vi "LCd.vi"() -> ()   [LabVIEW 2017]
panel:
  in  "String":string
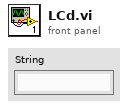
[diagram p1: front panel]
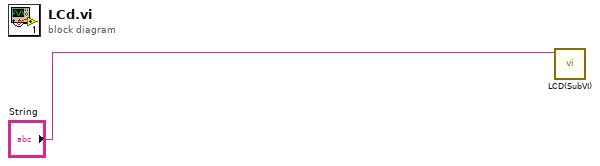
[diagram p0: block diagram]
diagram:
  n1 = call "LCD(SubVI).vi"("String"="String") -> ()  [unwired: 11 in]
